vi "U02453.vi"(1 "R (Ohm)":dbl=4203.0 format="%.5f") -> (0 "T (K)":dbl=0.29275308045912907 format="%.6f")   [LabVIEW 2018]
panel:
  in  "high range":T1={"ZL"=3.06751515602, "1"=18.744547, "2"=-19.474411, "3"=5.393362, "4"=-1.085942, "5"=0.267525, "6"=-0.047507, "7"=0.002563, "8"=-0.00811, "9"=0.0, "ZU"=3.18891164814} {"ZU" format="%#_12g"; "ZL" format="%#_14g"; "1" format="%#_14g"; "2" format="%#_14g"; "3" format="%#_14g"; "4" format="%#_14g"; "5" format="%#_14g"; "6" format="%#_14g"; "7" format="%#_14g"; "8" format="%#_14g"; "9" format="%#_14g"}
  in  "middle range":T1={"ZL"=3.17551397063, "1"=1.64712, "2"=-1.9920665, "3"=0.885108, "4"=-0.336273, "5"=0.113052, "6"=-0.032739, "7"=0.005671, "8"=0.0, "9"=0.0, "ZU"=3.38948858335} {"ZU" format="%#_12g"; "ZL" format="%#_14g"; "1" format="%#_14g"; "2" format="%#_14g"; "3" format="%#_14g"; "4" format="%#_14g"; "5" format="%#_14g"; "6" format="%#_14g"; "7" format="%#_14g"; "8" format="%#_14g"; "9" format="%#_14g"}
  out "Z":dbl
  out "k":dbl
  in  "low range":T1={"ZL"=3.34987560629, "1"=0.131724, "2"=-0.170454, "3"=0.075643, "4"=-0.027979, "5"=0.009206, "6"=-0.00238, "7"=0.00056, "8"=-8.3e-05, "9"=-0.000211, "ZU"=3.83157545445} {"ZU" format="%#_12g"; "ZL" format="%#_14g"; "1" format="%#_14g"; "2" format="%#_14g"; "3" format="%#_14g"; "4" format="%#_14g"; "5" format="%#_14g"; "6" format="%#_14g"; "7" format="%#_14g"; "8" format="%#_14g"; "9" format="%#_14g"}
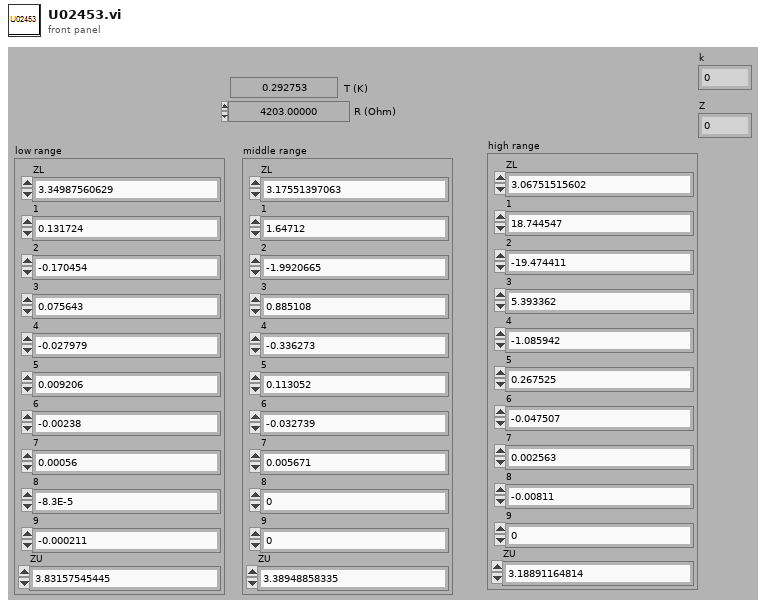
[diagram p1: front panel]
types:
  T1 = cluster{"ZL":dbl, "1":dbl, "2":dbl, "3":dbl, "4":dbl, "5":dbl, "6":dbl, "7":dbl, "8":dbl, "9":dbl, "ZU":dbl}
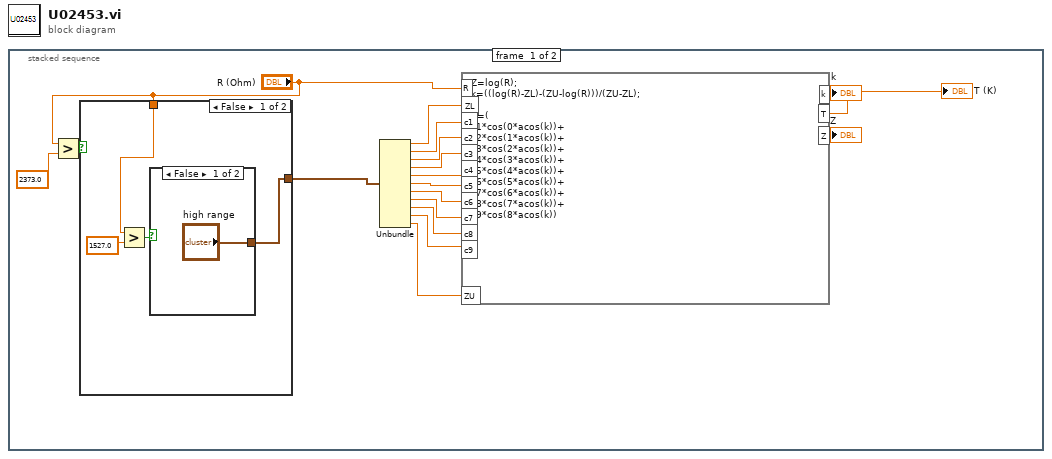
[diagram p0: block diagram]
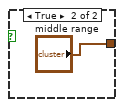
[diagram p2: hidden frame]
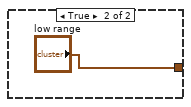
[diagram p3: hidden frame]
diagram:
  n1 = stacked-sequence {
    frame #0 {
      n2 = Greater?(x="R (Ohm)", y=2373.0) -> (0:w3:bool)
      n3 = case shown="False" w3 {
        tunnel: [w22 "low range"] -> w4
        tunnel: "R (Ohm)" -> [w20 _]
        frame False {
          n4 = Greater?(x=w20, y=1527.0) -> (0:w21:bool)
          n5 = case shown="False" w21 {
            tunnel: ["high range" "middle range"] -> w22
            frame False {
            }
            frame True {
            }
          }
        }
        frame True {
        }
      }
      n6 = Unbundle(w4) -> ("ZL"=w8:dbl, "1"=w9:dbl, "2"=w10:dbl, "3"=w11:dbl, "4"=w12:dbl, "5"=w13:dbl, "6"=w14:dbl, "7"=w15:dbl, "8"=w16:dbl, "9"=w17:dbl, "ZU"=w7:dbl)
      n7 = formula code="Z=log(R);\nk=((log(R)-ZL)-(ZU-log(R)))/(ZU-ZL);\n\nT=(\nc1*cos(0*acos(k))+\nc2*cos(1*acos(k))+\nc3*cos(2*acos(k))+\nc4*cos(3*acos(k))+\nc5*cos(4*acos(k))+\nc6*cos(5*acos(k))+\nc7*cos(6*acos(k))+\nc8*cos(7*acos(k))+\nc9*cos(8*acos(k))\n);"("R"="R (Ohm)", "ZL"=w8, "c1"=w9, "c2"=w10, "c3"=w11, "c4"=w12, "c5"=w13, "c6"=w14, "c7"=w15, "c8"=w16, "c9"=w17, "ZU"=w7) -> ("T"=→"T (K)":dbl, "k"=→"k":dbl, "Z"=→"Z":dbl)
    }
    frame #1 {
    }
  }
